vi "Webcam example.vi"(8 "error in (no error)":errorcluster) -> (0 "error out":errorcluster)   [LabVIEW 2012]
doc: "VI for streaming video from a webcam and show the temperature.\nBased on LibVLC.dll (http://www.videolan.org/) , needs an installation of this software to run.\nThe portable version of VLC is attached to the project"
uses:
  Controls-Webcam/VLC Var.ctl
  SubVIs-Webcam/subs/StartVideo PictureBox.vi
  System.Windows.Forms
panel:
  out "temporal error":errorcluster
  in  "VLC Variables In":T1
  in  "Subtitles":bool
  in  "Snap Shot Path":path=path "C:/DeleteMe/test.png"
  in  "Snapshot":bool
  in  "PictureBox":refnum<k24>(container)
  in  "Exit":bool
  # "C:\\Program Files (x86)\\VideoLAN\\VLC\\libvlc.dll"
  # "C:\\Archivos de programa\\VideoLAN\\VLC\\libvlc.dll"
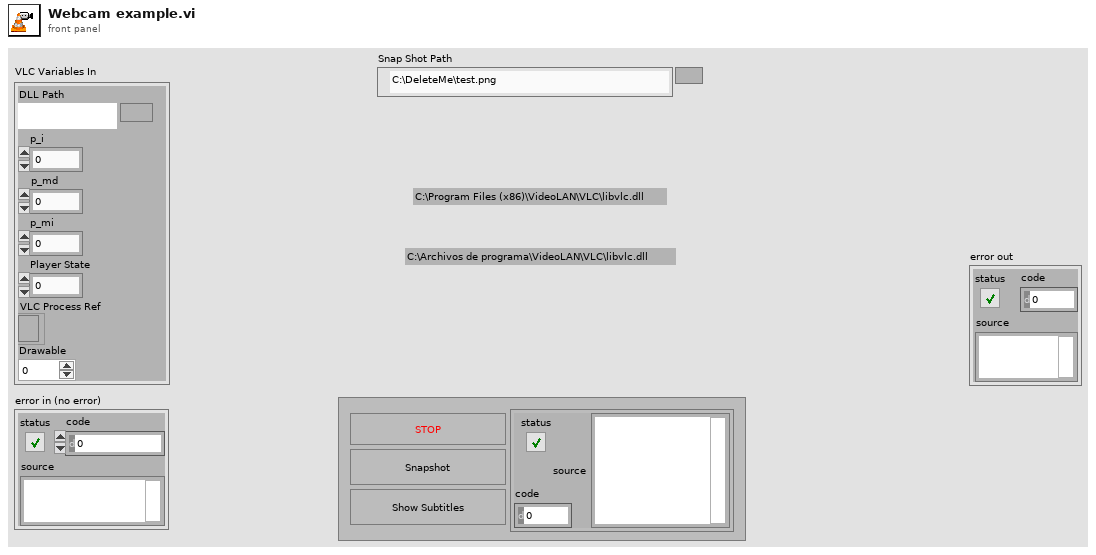
[diagram p1: front panel]
types:
  T1 = typedef "VLC Var.ctl" = cluster{"DLL Path":path, "p_i":i32, "p_md":i32, "p_mi":i32, "Player State":i32, "VLC Process Ref":refnum<k24>, "Drawable":i32}
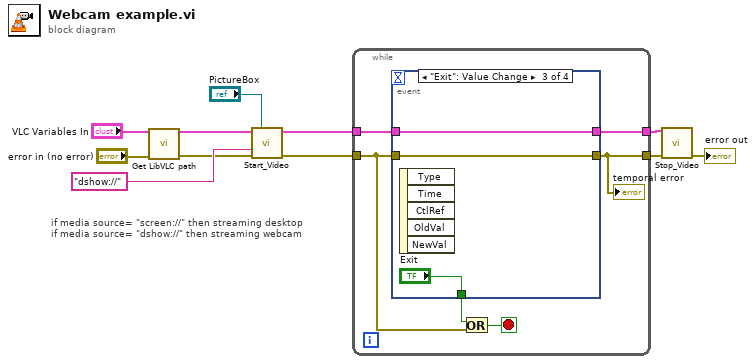
[diagram p0: block diagram]
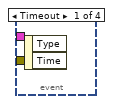
[diagram p2: hidden frame]
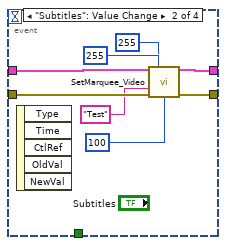
[diagram p3: hidden frame]
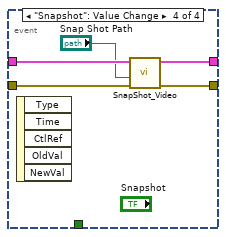
[diagram p4: hidden frame]
diagram:
  # "if media source= \"screen://\" then streaming desktop\nif media source= \"dshow://\" then streaming webcam"
  n1 = call "Get LibVLC path.vi"("VLC Variables In"="VLC Variables In", "error in (no error)"="error in (no error)") -> ("VLC Variables Out"=w1:T1, "error out"=w7:errorcluster)  [unwired: 12 in]
  n2 = call-poly "Start_Video.vi"("VLC Variables In"=w1, "PictureBox"="PictureBox", "Media Source"="dshow://", "error in (no error)"=w7) -> ("VLC Variables Out"=w9:T1, "error out"=w3:errorcluster)  [unwired: 10 in]
  n3 = while {
    tunnel: w9 -> [w14]
    tunnel: [w15] -> w5
    tunnel: [w12] -> w4
    tunnel: w3 -> [w13]
    stop <- w17 stop-if-true
    n4 = event shown="[2] \"Exit\": Value Change" {
      selector: _ -> [_ _ _ _]
      dyn-events: _ -> [_ _ _ _]
      timeout: _ -> [_ _ _ _]
      tunnel: [_ _ "Exit" _] -> w16
      tunnel: [_ w25 w27 w33] -> w12
      tunnel: [_ w18 w26 w32] -> w15
      tunnel: w14 -> [_ w23 w26 w31]
      tunnel: w13 -> [_ w22 w27 w30]
      event Timeout {
        n5 = event-data() -> ()  [unwired: 1 in, 2 out]
      }
      event "Subtitles": Value Change {
        n6 = event-data() -> ()  [unwired: 1 in, 5 out]
        n7 = call "SetMarquee_Video.vi"("VLC Variables"=w23, "x-coordinate"=255 ("opacity"), "y-coordinate"=100, "String"="Test", "error in (no error)"=w22, "opacity"=255 ("x-coordinate")) -> ("VLC Variables Out"=w18:T1, "error out"=w25:errorcluster)  [unwired: 8 in]
      }
      event "Exit": Value Change {
        n8 = event-data() -> ()  [unwired: 1 in, 5 out]
      }
      event "Snapshot": Value Change {
        n9 = event-data() -> ()  [unwired: 1 in, 5 out]
        n10 = call "SnapShot_Video.vi"("error in (no error)"=w30, "Snnp Shot Path"="Snap Shot Path", "VLC Variables"=w31) -> ("error out"=w33:errorcluster, "VLC Variables Out"=w32:T1)  [unwired: 7 in]
      }
    }
    "temporal error" <- w12
    n11 = Or(x=w16, y=w13) -> (x .or. y?=w17:bool)
  }
  n12 = call "Stop_Video.vi"("VLC Variables In"=w5, "error in (no error)"=w4) -> ("error out"=→"error out":errorcluster)  [unwired: 13 in]
